vi "Main.vi"() -> ()   [LabVIEW 2014]
uses:
  MainDataTypedef.ctl
  <vilib>/Utility/sysdir.llb/System Directory Type.ctl
panel:
  out "UpdateValue":bool
  out "Cluster":T1 {"SetValueCluster"."Ring 0" items=["AA", "BB", "CC"]; "SetValueCluster"."Ring 1" items=["AA", "BB", "CC"]; "SetValueCluster"."Ring 2" items=["AA", "BB", "CC"]; "SetValueCluster"."Ring 3" items=["AA", "BB", "CC"]; "SetValueCluster"."Ring 4" items=["AA", "BB", "CC"]; "SetValueCluster"."Ring 5" items=["AA", "BB", "CC"]; "SetValueCluster"."Ring 6" items=["AA", "BB", "CC"]; "SetValueCluster"."Ring 7" items=["AA", "BB", "CC"]; "SetValueCluster"."Ring 8" items=["AA", "BB", "CC"]; "SetValueCluster"."Ring 9" items=["AA", "BB", "CC"]; "SetValueCluster"."Ring 10" items=["AA", "BB", "CC"]; "SetValueCluster"."Ring 11" items=["AA", "BB", "CC"]; "SetValueCluster"."Ring 12" items=["AA", "BB", "CC"]}
  in  "Load":bool
  in  "Save":bool
  out "INIT":bool
  in  "Ring 12":u16(ring) items=["AA", "BB", "CC"]
  in  "String 12":string
  in  "Switch 12":bool
  in  "Numeric 12":dbl
  in  "Ring 11":u16(ring) items=["AA", "BB", "CC"]
  in  "Ring 10":u16(ring) items=["AA", "BB", "CC"]
  in  "Ring 9":u16(ring) items=["AA", "BB", "CC"]
  in  "Ring 8":u16(ring) items=["AA", "BB", "CC"]
  in  "Ring 7":u16(ring) items=["AA", "BB", "CC"]
  in  "Ring 6":u16(ring) items=["AA", "BB", "CC"]
  in  "Ring 5":u16(ring) items=["AA", "BB", "CC"]
  in  "Ring 4":u16(ring) items=["AA", "BB", "CC"]
  in  "Ring 3":u16(ring) items=["AA", "BB", "CC"]
  in  "Ring 2":u16(ring) items=["AA", "BB", "CC"]
  in  "Ring 1":u16(ring) items=["AA", "BB", "CC"]
  in  "String 11":string
  in  "String 10":string
  in  "String 9":string
  in  "String 8":string
  in  "String 7":string
  in  "String 6":string
  in  "String 5":string
  in  "String 4":string
  in  "String 3":string
  in  "String 2":string
  in  "String 1":string
  in  "Switch 11":bool
  in  "Switch 10":bool
  in  "Switch 9":bool
  in  "Switch 8":bool
  in  "Switch 7":bool
  in  "Switch 6":bool
  in  "Switch 5":bool
  in  "Switch 4":bool
  in  "Switch 3":bool
  in  "Switch 2":bool
  in  "Switch 1":bool
  in  "Numeric 11":dbl
  in  "Numeric 10":dbl
  in  "Numeric 9":dbl
  in  "Numeric 8":dbl
  in  "Numeric 7":dbl
  in  "Numeric 6":dbl
  in  "Numeric 5":dbl
  in  "Numeric 4":dbl
  in  "Numeric 3":dbl
  in  "Numeric 2":dbl
  in  "Numeric 1":dbl
  in  "Ring 0":u16(ring) items=["AA", "BB", "CC"]
  in  "String 0":string
  in  "Switch 0":bool
  in  "Numeric 0":dbl
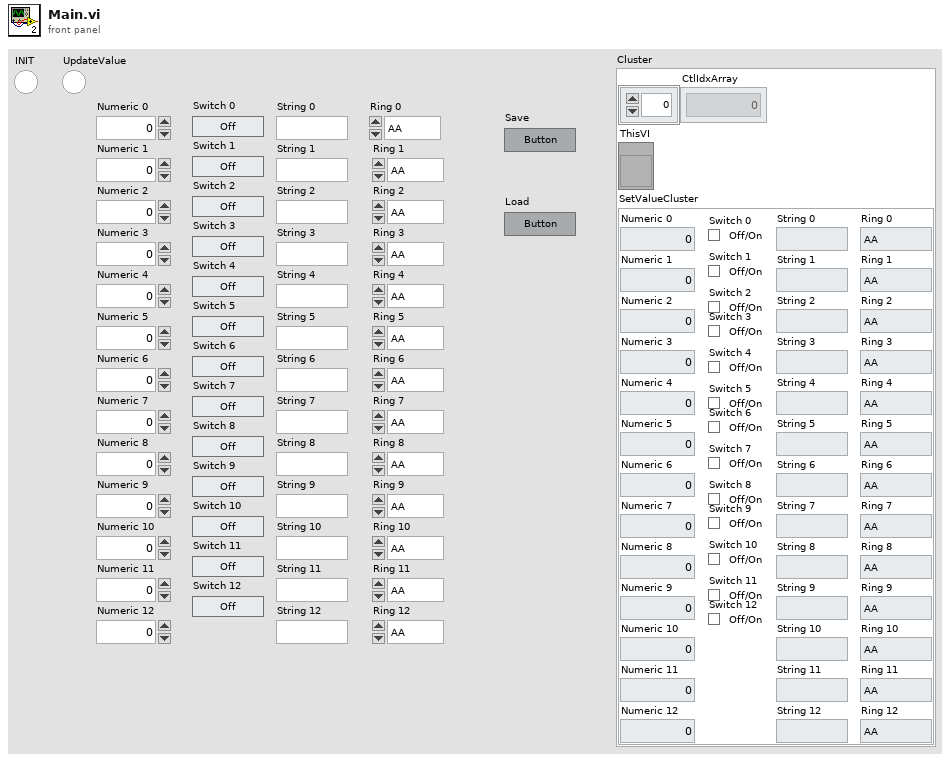
[diagram p1: front panel]
types:
  T1 = typedef "MainDataTypedef.ctl" = cluster{"CtlIdxArray":i32[], "ThisVI":refnum<vi>, "SetValueCluster":cluster{"Numeric 0":dbl, "Numeric 1":dbl, "Numeric 2":dbl, "Numeric 3":dbl, "Numeric 4":dbl, "Numeric 5":dbl, "Numeric 6":dbl, "Numeric 7":dbl, "Numeric 8":dbl, "Numeric 9":dbl, "Numeric 10":dbl, "Numeric 11":dbl, "Numeric 12":dbl, "Switch 0":bool, "Switch 1":bool, "Switch 2":bool, "Switch 3":bool, "Switch 4":bool, "Switch 5":bool, "Switch 6":bool, "Switch 7":bool, "Switch 8":bool, "Switch 9":bool, "Switch 10":bool, "Switch 11":bool, "Switch 12":bool, "String 0":string, "String 1":string, "String 2":string, "String 3":string, "String 4":string, "String 5":string, "String 6":string, "String 7":string, "String 8":string, "String 9":string, "String 10":string, "String 11":string, "String 12":string, "Ring 0":u16, "Ring 1":u16, "Ring 2":u16, "Ring 3":u16, "Ring 4":u16, "Ring 5":u16, "Ring 6":u16, "Ring 7":u16, "Ring 8":u16, "Ring 9":u16, "Ring 10":u16, "Ring 11":u16, "Ring 12":u16}}
  T2 = cluster{"Numeric 0":dbl, "Numeric 1":dbl, "Numeric 2":dbl, "Numeric 3":dbl, "Numeric 4":dbl, "Numeric 5":dbl, "Numeric 6":dbl, "Numeric 7":dbl, "Numeric 8":dbl, "Numeric 9":dbl, "Numeric 10":dbl, "Numeric 11":dbl, "Numeric 12":dbl, "Switch 0":bool, "Switch 1":bool, "Switch 2":bool, "Switch 3":bool, "Switch 4":bool, "Switch 5":bool, "Switch 6":bool, "Switch 7":bool, "Switch 8":bool, "Switch 9":bool, "Switch 10":bool, "Switch 11":bool, "Switch 12":bool, "String 0":string, "String 1":string, "String 2":string, "String 3":string, "String 4":string, "String 5":string, "String 6":string, "String 7":string, "String 8":string, "String 9":string, "String 10":string, "String 11":string, "String 12":string, "Ring 0":u16, "Ring 1":u16, "Ring 2":u16, "Ring 3":u16, "Ring 4":u16, "Ring 5":u16, "Ring 6":u16, "Ring 7":u16, "Ring 8":u16, "Ring 9":u16, "Ring 10":u16, "Ring 11":u16, "Ring 12":u16}
  T3 = typedef "System Directory Type.ctl" = i32
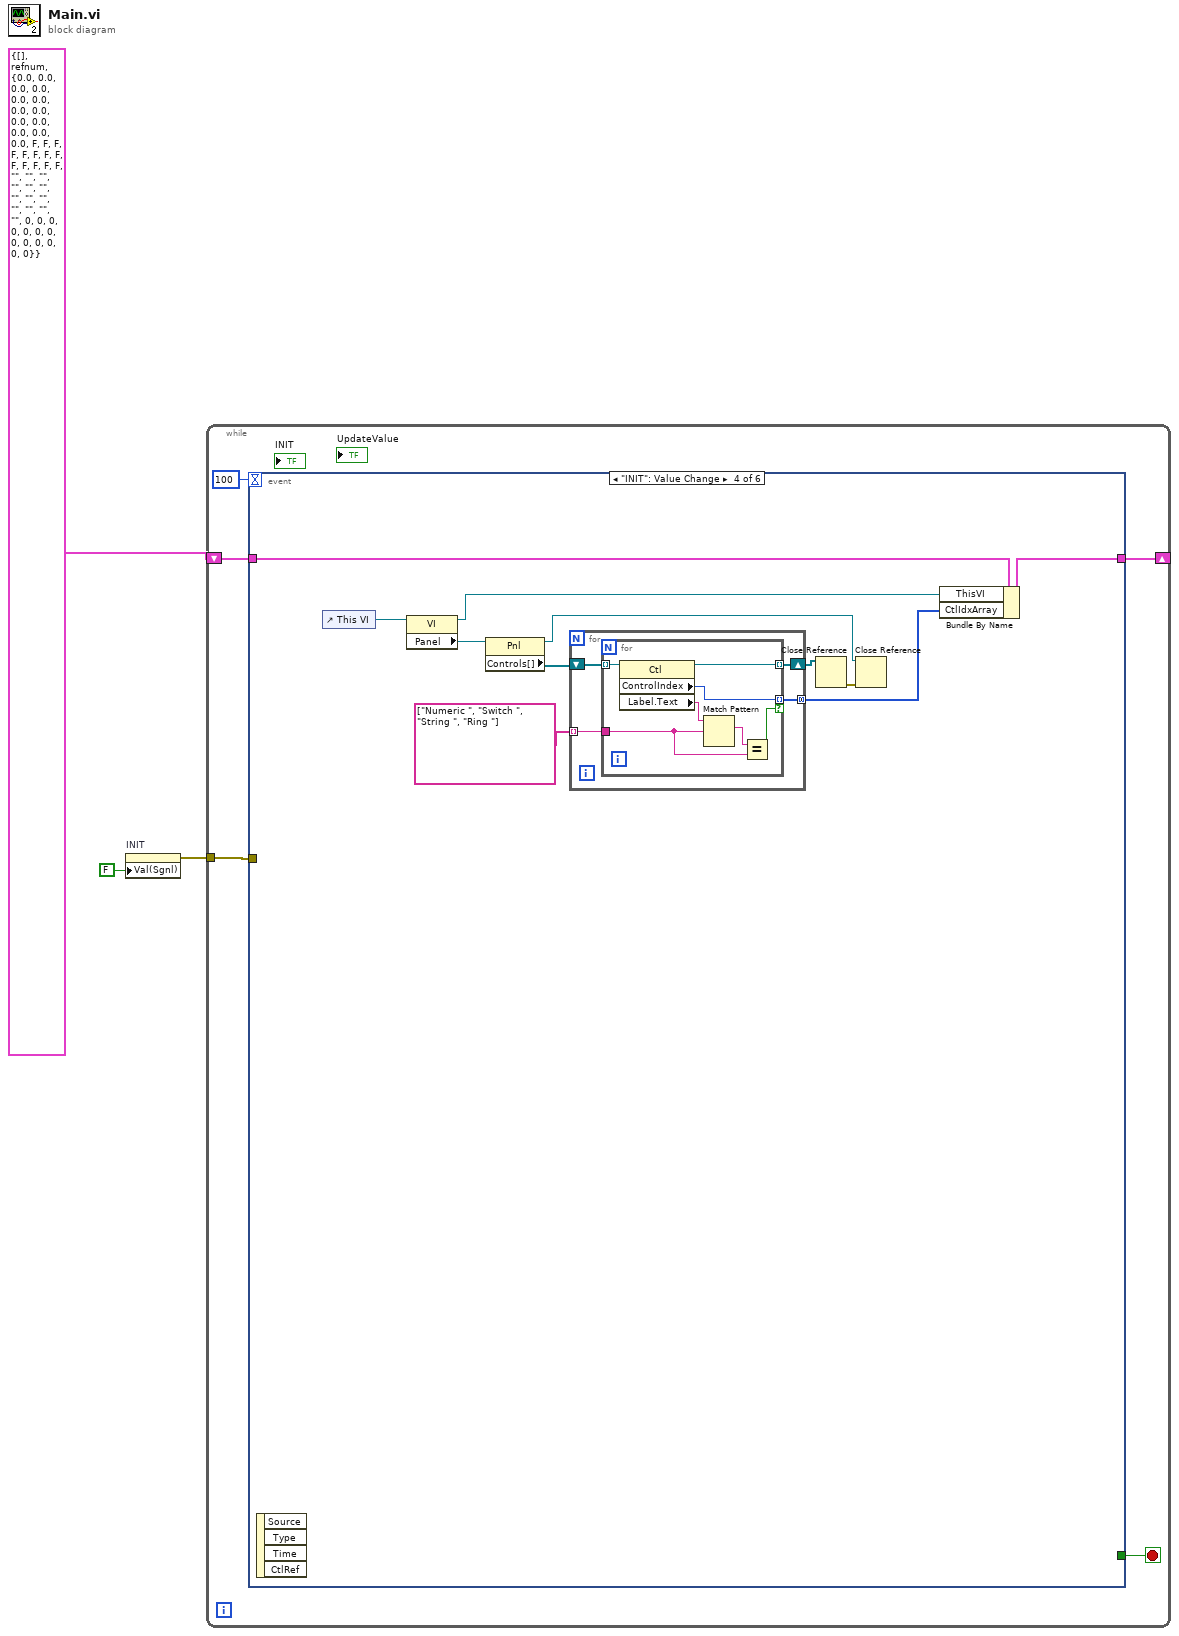
[diagram p0: block diagram]
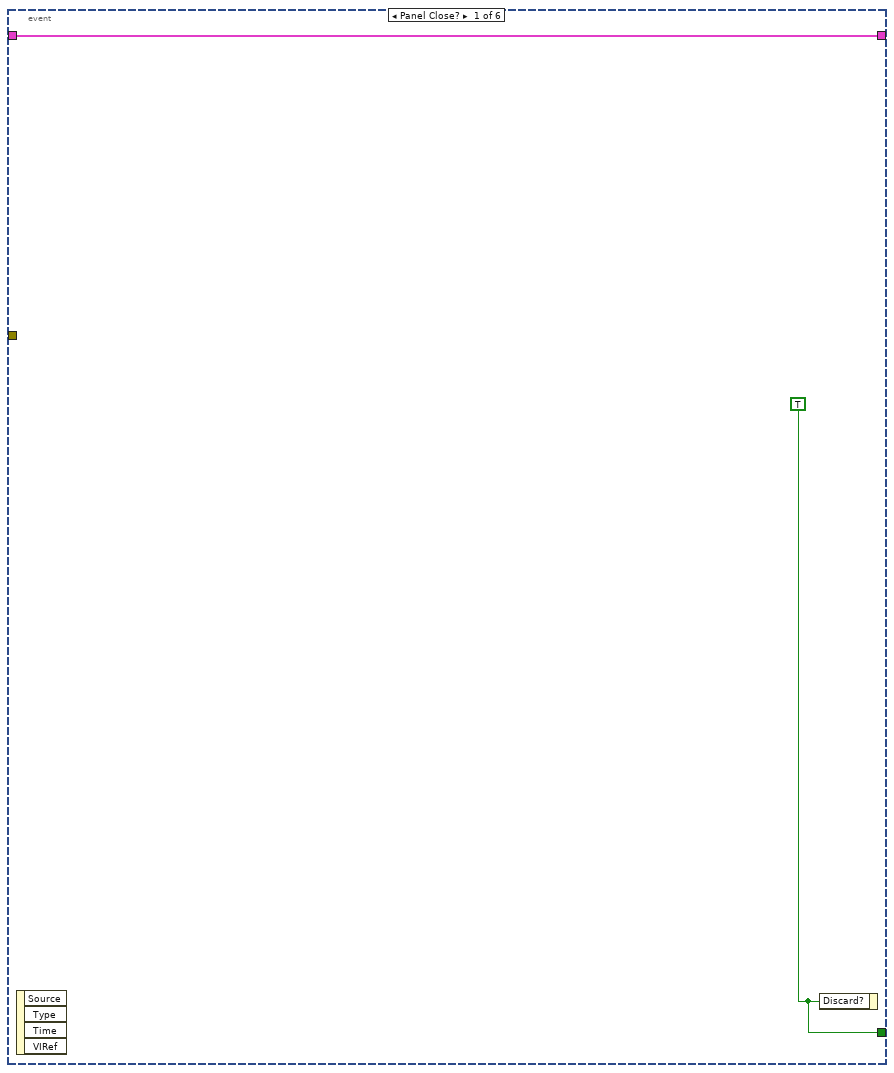
[diagram p2: hidden frame]
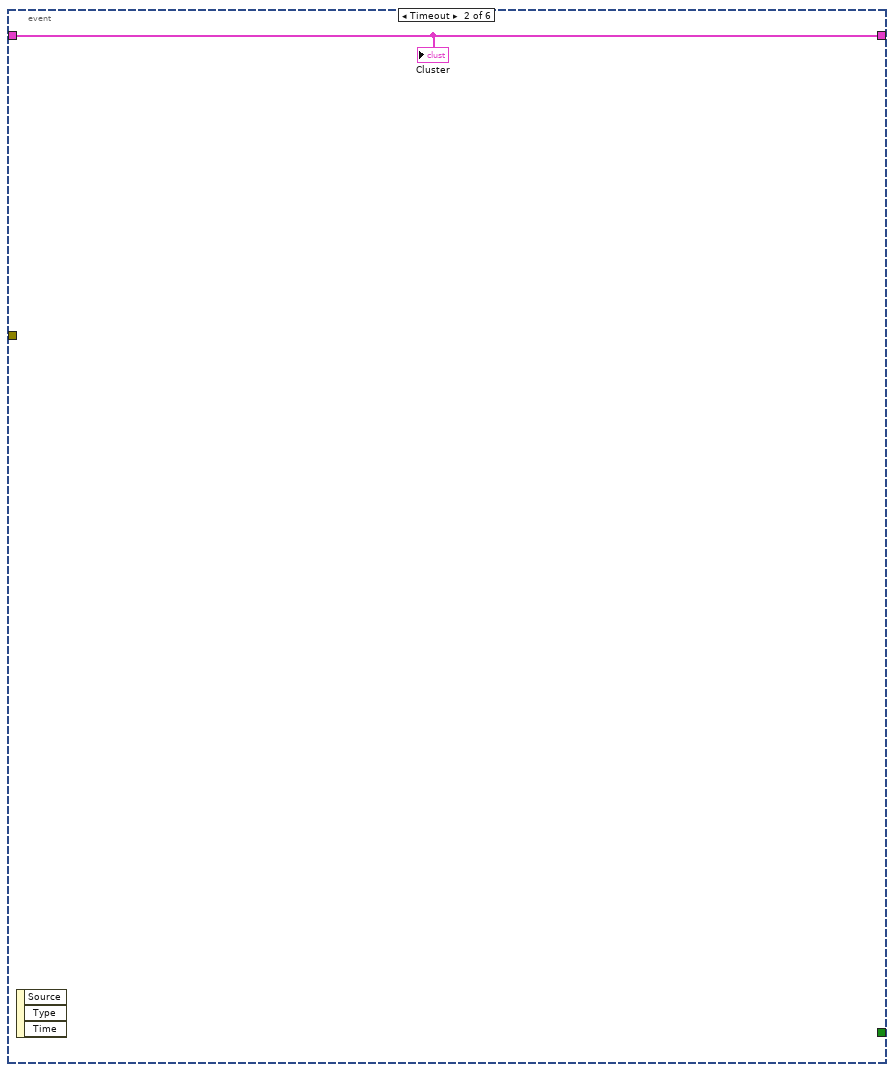
[diagram p3: hidden frame]
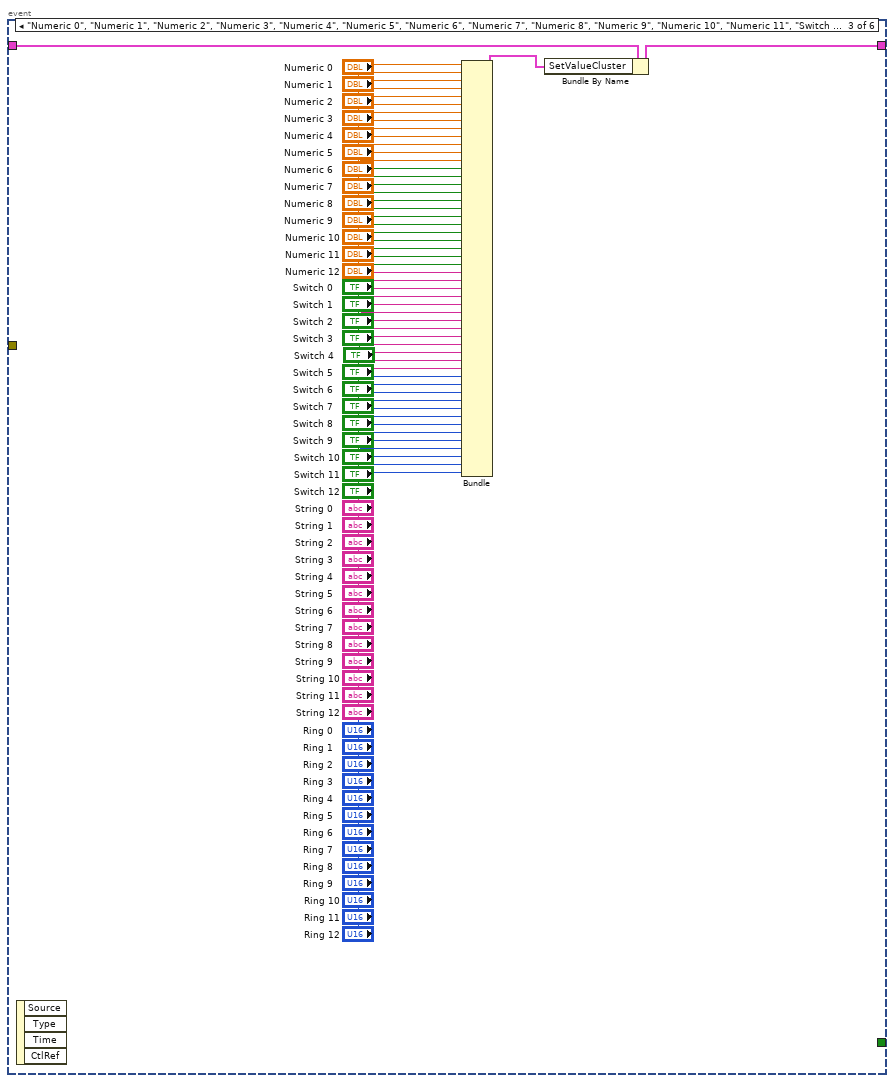
[diagram p4: hidden frame]
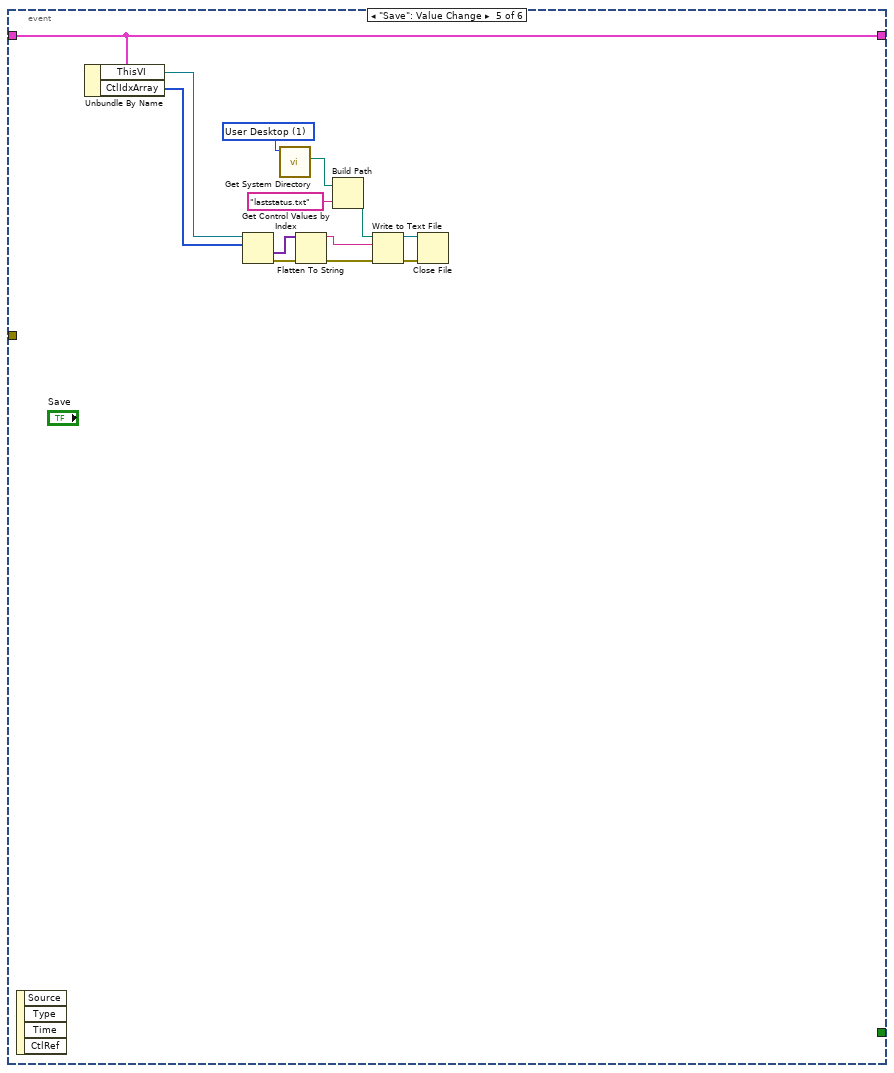
[diagram p5: hidden frame]
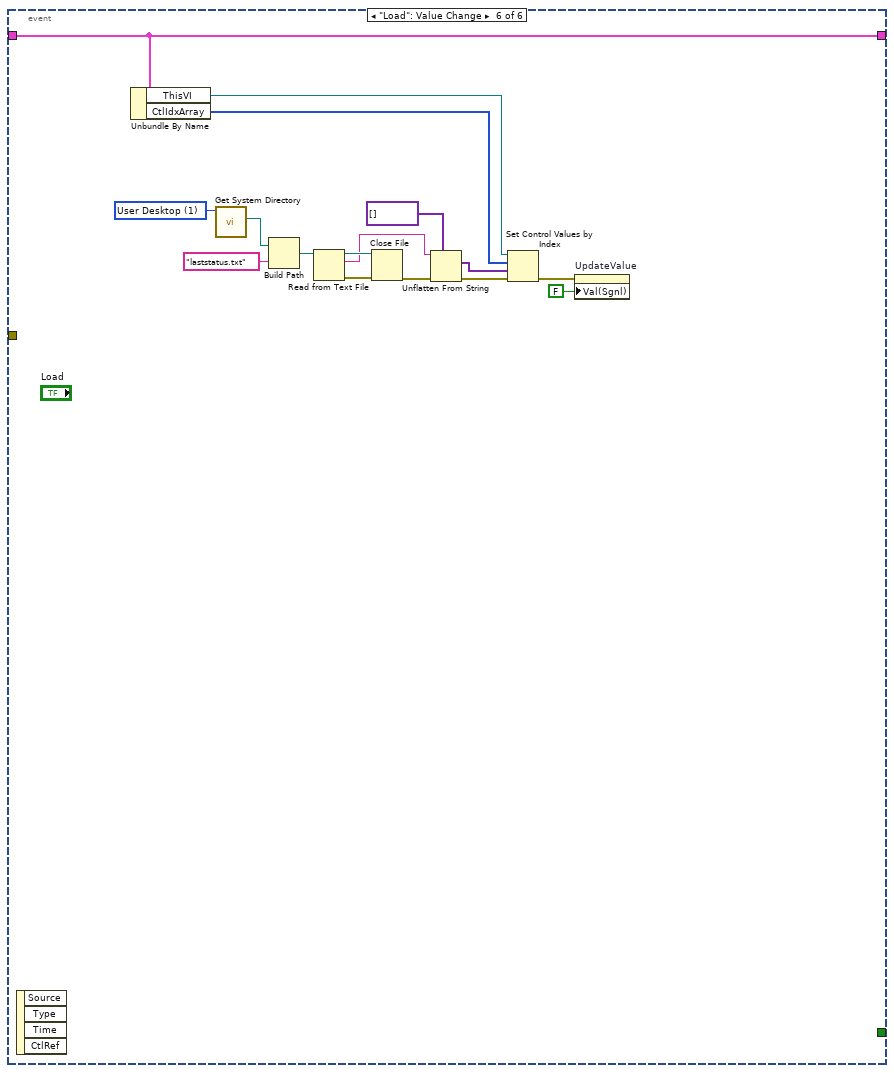
[diagram p6: hidden frame]
diagram:
  n1 = property on="INIT" class="Bool (strict)"("Val(Sgnl)"=FALSE ("Value (Signaling)")) -> (error out=w3:errorcluster)  [unwired: 2 in, 1 out]
  n2 = while {
    shift-right: [w6] -> _
    shift-left: T1 {"CtlIdxArray"=[], "ThisVI"=refnum, "SetValueCluster"={"Numeric 0"=0.0, "Numeric 1"=0.0, "Numeric 2"=0.0, "Numeric 3"=0.0, "Numeric 4"=0.0, "Numeric 5"=0.0, "Numeric 6"=0.0, "Numeric 7"=0.0, "Numeric 8"=0.0, "Numeric 9"=0.0, "Numeric 10"=0.0, "Numeric 11"=0.0, "Numeric 12"=0.0, "Switch 0"=FALSE, "Switch 1"=FALSE, "Switch 2"=FALSE, "Switch 3"=FALSE, "Switch 4"=FALSE, "Switch 5"=FALSE, "Switch 6"=FALSE, "Switch 7"=FALSE, "Switch 8"=FALSE, "Switch 9"=FALSE, "Switch 10"=FALSE, "Switch 11"=FALSE, "Switch 12"=FALSE, "String 0"="", "String 1"="", "String 2"="", "String 3"="", "String 4"="", "String 5"="", "String 6"="", "String 7"="", "String 8"="", "String 9"="", "String 10"="", "String 11"="", "String 12"="", "Ring 0"=0, "Ring 1"=0, "Ring 2"=0, "Ring 3"=0, "Ring 4"=0, "Ring 5"=0, "Ring 6"=0, "Ring 7"=0, "Ring 8"=0, "Ring 9"=0, "Ring 10"=0, "Ring 11"=0, "Ring 12"=0}} ("Cluster") -> [w5]
    tunnel: w3 -> [w7]
    stop <- w8 stop-if-true
    n3 = event shown="[3] \"INIT\": Value Change" {
      selector: _ -> [_ _ _ _ _ _]
      dyn-events: _ -> [_ _ _ _ _ _]
      timeout: 100 -> [_ _ _ _ _ _]
      tunnel: [w10 _ _ _ _ _] -> w8
      tunnel: w7 -> [_ _ _ _ _ _]
      tunnel: [w9 w11 w65 w74 w101 w108] -> w6
      tunnel: w5 -> [w9 w11 w66 w76 w101 w108]
      event Panel Close? {
        w10 = TRUE ("Discard?")
        n4 = event-data() -> ()  [unwired: 1 in, 4 out]
        n5 = event-data("Discard?"=w10) -> ()  [unwired: 1 in, 1 out]
      }
      event Timeout {
        n6 = event-data() -> ()  [unwired: 1 in, 3 out]
        "Cluster" <- w11
      }
      event "Numeric 0", "Numeric 1", "Numeric 2", "Numeric 3", "Numeric 4", "Numeric 5", "Numeric 6", "Numeric 7", "Numeric 8", "Numeric 9", "Numeric 10", "Numeric 11", "Switch 0", "Switch 1", "Switch 2", "Switch 3", "Switch 4", "Switch 5", "Switch 6", "Switch 7", "Switch 8", "Switch 9", "Switch 10", "Switch 11", "String 0", "String 1", "String 2", "String 3", "String 4", "String 5", "String 6", "String 7", "String 8", "String 9", "String 10", "String 11", "Ring 0", "Ring 1", "Ring 2", "Ring 3", "Ring 4", "Ring 5", "Ring 6", "Ring 7", "Ring 8", "Ring 9", "Ring 10", "Ring 11", "UpdateValue": Value Change {
        n7 = event-data() -> ()  [unwired: 1 in, 4 out]
        n8 = Bundle("Numeric 0"="Numeric 0", "Numeric 1"="Numeric 1", "Numeric 2"="Numeric 2", "Numeric 3"="Numeric 3", "Numeric 4"="Numeric 4", "Numeric 5"="Numeric 5", "Numeric 6"="Numeric 6", "Numeric 7"="Numeric 7", "Numeric 8"="Numeric 8", "Numeric 9"="Numeric 9", "Numeric 10"="Numeric 10", "Numeric 11"="Numeric 11", "Numeric 12"="Numeric 12", "Switch 0"="Switch 0", "Switch 1"="Switch 1", "Switch 2"="Switch 2", "Switch 3"="Switch 3", "Switch 4"="Switch 4", "Switch 5"="Switch 5", "Switch 6"="Switch 6", "Switch 7"="Switch 7", "Switch 8"="Switch 8", "Switch 9"="Switch 9", "Switch 10"="Switch 10", "Switch 11"="Switch 11", "Switch 12"="Switch 12", "String 0"="String 0", "String 1"="String 1", "String 2"="String 2", "String 3"="String 3", "String 4"="String 4", "String 5"="String 5", "String 6"="String 6", "String 7"="String 7", "String 8"="String 8", "String 9"="String 9", "String 10"="String 10", "String 11"="String 11", "String 12"="String 12", "Ring 0"="Ring 0", "Ring 1"="Ring 1", "Ring 2"="Ring 2", "Ring 3"="Ring 3", "Ring 4"="Ring 4", "Ring 5"="Ring 5", "Ring 6"="Ring 6", "Ring 7"="Ring 7", "Ring 8"="Ring 8", "Ring 9"="Ring 9", "Ring 10"="Ring 10", "Ring 11"="Ring 11", "Ring 12"="Ring 12") -> (w12:T2)  [unwired: 1 in]
        n9 = Bundle By Name(cluster=w66, "SetValueCluster"=w12) -> (w65:T1)
      }
      event "INIT": Value Change {
        n10 = event-data() -> ()  [unwired: 1 in, 4 out]
        n11 = control-ref of="This VI"() -> (w72:refnum<vi>)
        n12 = property class="VI"(reference=w72) -> (reference out=w70:refnum<vi>, "Panel"=w71:refnum<vi>)  [unwired: 1 in, 1 out]
        n13 = property class="Pnl"(reference=w71) -> (reference out=w67:refnum<vi>, "Controls[]"=w77:refnum<vi>[])  [unwired: 1 in, 1 out]
        n14 = for {
          tunnel: string[] ["Numeric ", "Switch ", "String ", "Ring "] ("regular expression") -> [w80] mode=indexing
          tunnel: [w79] -> w73 mode=concatenating
          shift-right: [w78] -> w69
          shift-left: w77 -> [w81]
          n15 = for {
            tunnel: w81 -> [w88] mode=indexing
            tunnel: w80 -> [w87]
            tunnel: [w83] -> w79 mode=indexing if=w84
            tunnel: [w82] -> w78 mode=indexing
            n16 = property class="Ctl"(reference=w88) -> (reference out=w82:refnum<vi>, "ControlIndex"=w83:i32, "Label.Text"=w86:string)  [unwired: 1 in, 1 out]
            n17 = Match Pattern(string=w86, regular expression=w87) -> (match substring=w85:string)  [unwired: 1 in, 3 out]
            n18 = Equal?(x=w85, y=w87) -> (x = y?=w84:bool)
          }
        }
        n19 = Close Reference(reference=w69) -> (error out=w68:errorcluster)  [unwired: 1 in]
        n20 = Close Reference(reference=w67, error in (no error)=w68) -> ()  [unwired: 1 out]
        n21 = Bundle By Name(cluster=w76, "ThisVI"=w70, "CtlIdxArray"=w73) -> (w74:T1)
      }
      event "Save": Value Change {
        w97 = T3 1 items=["User Home"=0, "User Desktop"=1, "User Documents"=2, "User Application Data"=3, "User Preferences"=4, "User Temporary"=5, "Public Documents"=6, "Public Application Data"=7, "Public Preferences"=8, "Public Cache"=13, "System Core Libraries"=9, "System Installed Libraries"=10, "Application Files"=11, "Boot Volume Root"=12] ("system directory type")
        n22 = event-data() -> ()  [unwired: 1 in, 4 out]
        n23 = Unbundle By Name(w101) -> ("ThisVI"=w98:refnum<vi>, "CtlIdxArray"=w100:i32[])
        n24 = Get Control Values by Index(0:w98, 1:w100) -> (10:w99:variant[], 11:w90:errorcluster)  [unwired: 1 in]
        n25 = call <vilib>:"Get System Directory.vi"("system directory type"=w97) -> ("system directory"=w96:path)  [unwired: 10 in]
        n26 = Flatten To String(anything=w99, error in (no error)=w90) -> (data string=w93:string, error out=w89:errorcluster)  [unwired: 2 in, 1 out]
        n27 = Build Path(base path=w96, name or relative path="laststatus.txt") -> (appended path=w94:path)
        n28 = Write to Text File(file (use dialog)=w94, text=w93, error in=w89) -> (refnum out=w92:refnum<file>, error out=w91:errorcluster)  [unwired: 1 in, 1 out]
        n29 = Close File(refnum=w92, error in=w91) -> ()  [unwired: 2 out]
      }
      event "Load": Value Change {
        w117 = T3 1 items=["User Home"=0, "User Desktop"=1, "User Documents"=2, "User Application Data"=3, "User Preferences"=4, "User Temporary"=5, "Public Documents"=6, "Public Application Data"=7, "Public Preferences"=8, "Public Cache"=13, "System Core Libraries"=9, "System Installed Libraries"=10, "Application Files"=11, "Boot Volume Root"=12] ("system directory type")
        n30 = event-data() -> ()  [unwired: 1 in, 4 out]
        n31 = Unbundle By Name(w108) -> ("ThisVI"=w107:refnum<vi>, "CtlIdxArray"=w106:i32[])
        n32 = call <vilib>:"Get System Directory.vi"("system directory type"=w117) -> ("system directory"=w116:path)  [unwired: 10 in]
        n33 = Build Path(base path=w116, name or relative path="laststatus.txt") -> (appended path=w114:path)
        n34 = Read from Text File(file (use dialog)=w114) -> (refnum out=w113:refnum<file>, text=w110:string, error out=w112:errorcluster)  [unwired: 3 in, 1 out]
        n35 = Close File(refnum=w113, error in=w112) -> (error out=w111:errorcluster)  [unwired: 1 out]
        n36 = Unflatten From String(type=variant[] [] ("data values"), binary string=w110, error in (no error)=w111) -> (value=w105:variant[], error out=w104:errorcluster)  [unwired: 2 in, 1 out]
        n37 = Set Control Values by Index(0:w107, 1:w106, 2:w105, 3:w104) -> (11:w103:errorcluster)
        n38 = property on="UpdateValue" class="Bool (strict)"(error in=w103, "Val(Sgnl)"=FALSE ("Value (Signaling)")) -> ()  [unwired: 1 in, 2 out]
      }
    }
  }
